vi "ControlNameEscape.vi"(10 "Escape Control Chars (true)":bool=TRUE, 11 "label":string) -> (3 "escaped string":string)   [LabVIEW 2021, in "SetGetControlValue.lvlib"]
uses:
  SetGetControlValue.lvlib
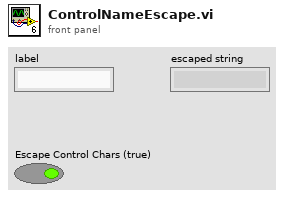
[diagram p1: front panel]
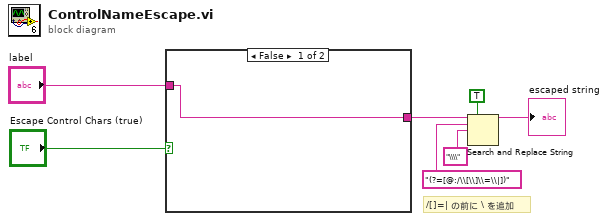
[diagram p0: block diagram]
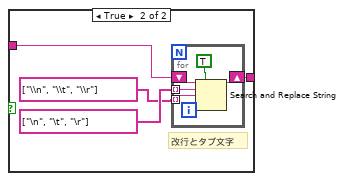
[diagram p2: hidden frame]
diagram:
  # "/[]=| の前に \\ を追加"
  n1 = case shown="False" "Escape Control Chars (true)" {
    tunnel: "label" -> [w8 w12]
    tunnel: [w8 w11] -> w2
    frame False {
    }
    frame True {
      # "改行とタブ文字"
      n2 = for {
        tunnel: string[] ["\n", "\t", "\r"] ("search string") -> [w17] mode=indexing
        tunnel: string[] ["\\n", "\\t", "\\r"] ("search string") -> [w16] mode=indexing
        shift-right: [w14] -> w11
        shift-left: w12 -> [w15]
        n3 = Search and Replace String(replace all?=TRUE ("replace all? (F)"), input string=w15, search string=w17, replace string=w16) -> (result string=w14:string)  [unwired: 4 in, 3 out]
      }
    }
  }
  n4 = Search and Replace String(replace all?=TRUE ("replace all? (F)"), input string=w2, search string="(?=[@:/\\[\\]\\=\\|])", replace string="\\\\" ("replace string (\"\")")) -> (result string=→"escaped string":string)  [unwired: 4 in, 3 out]
